vi "Draw Tree and set expand settings.vi"(8 "error in":errorcluster, 9 "Expanded Results?":bool, 10 "Tree Control Items":T1(array[cluster]), 11 "TreeControl in":refnum<vi>) -> (0 "error out":errorcluster)   [LabVIEW 2019, in "Panther Dashboard.lvlib"]
uses:
  Panther Dashboard.lvlib
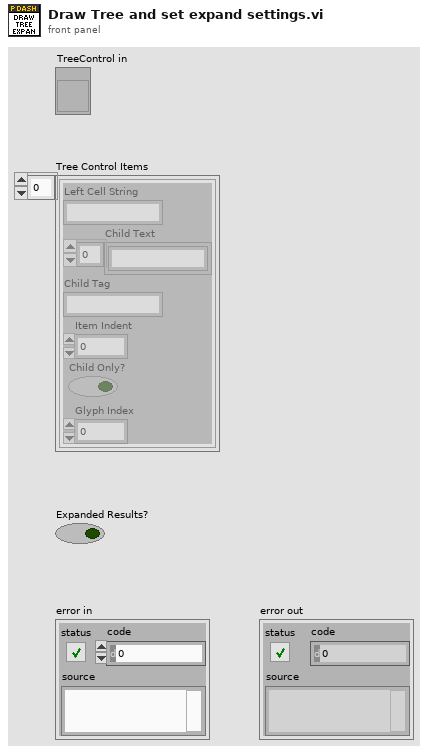
[diagram p1: front panel]
types:
  T1 = cluster{"Left Cell String":string, "Child Text":string[], "Child Tag":string, "Item Indent":i32, "Child Only?":bool, "Glyph Index":i32}[]
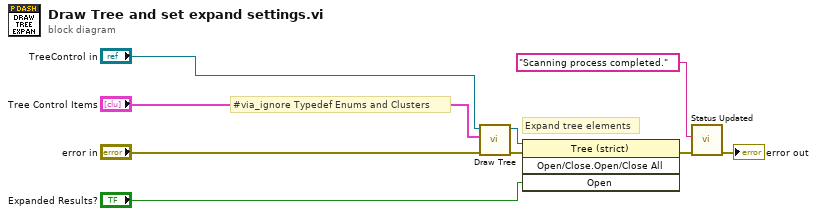
[diagram p0: block diagram]
diagram:
  # "Expand tree elements"
  # "#via_ignore Typedef Enums and Clusters"
  n1 = call "Draw Tree.vi"("error in"="error in", "Tree Control Items"="Tree Control Items", "TreeControl in"="TreeControl in") -> ("error out"=w9:errorcluster, "TreeControl out"=w4:refnum<vi>)  [unwired: 7 in]
  n2 = invoke class="Tree (strict)" method="Open/Close.Open/Close All"(reference=w4, error in=w9, "Open"="Expanded Results?") -> (error out=w7:errorcluster)  [unwired: 1 in, 3 out]
  n3 = call "Status Updated.vi"("error in (no error)"=w7, "Status"="Scanning process completed.") -> ("error out"=→"error out":errorcluster)  [unwired: 9 in]
